vi "IP SETTING.vi"() -> ()   [LabVIEW 2017]
uses:
  <vilib>/addons/database/Connection.llb/DB Tools Open Connec (String).vi
  Global/Global 1.vi
  <vilib>/addons/database/NI_Database_API.lvlib
panel:
  in  "SAVE":bool
  in  "Cluster":T1
  out "error out":errorcluster
  in  "error in (no error)":errorcluster
  in  "EXIT":bool
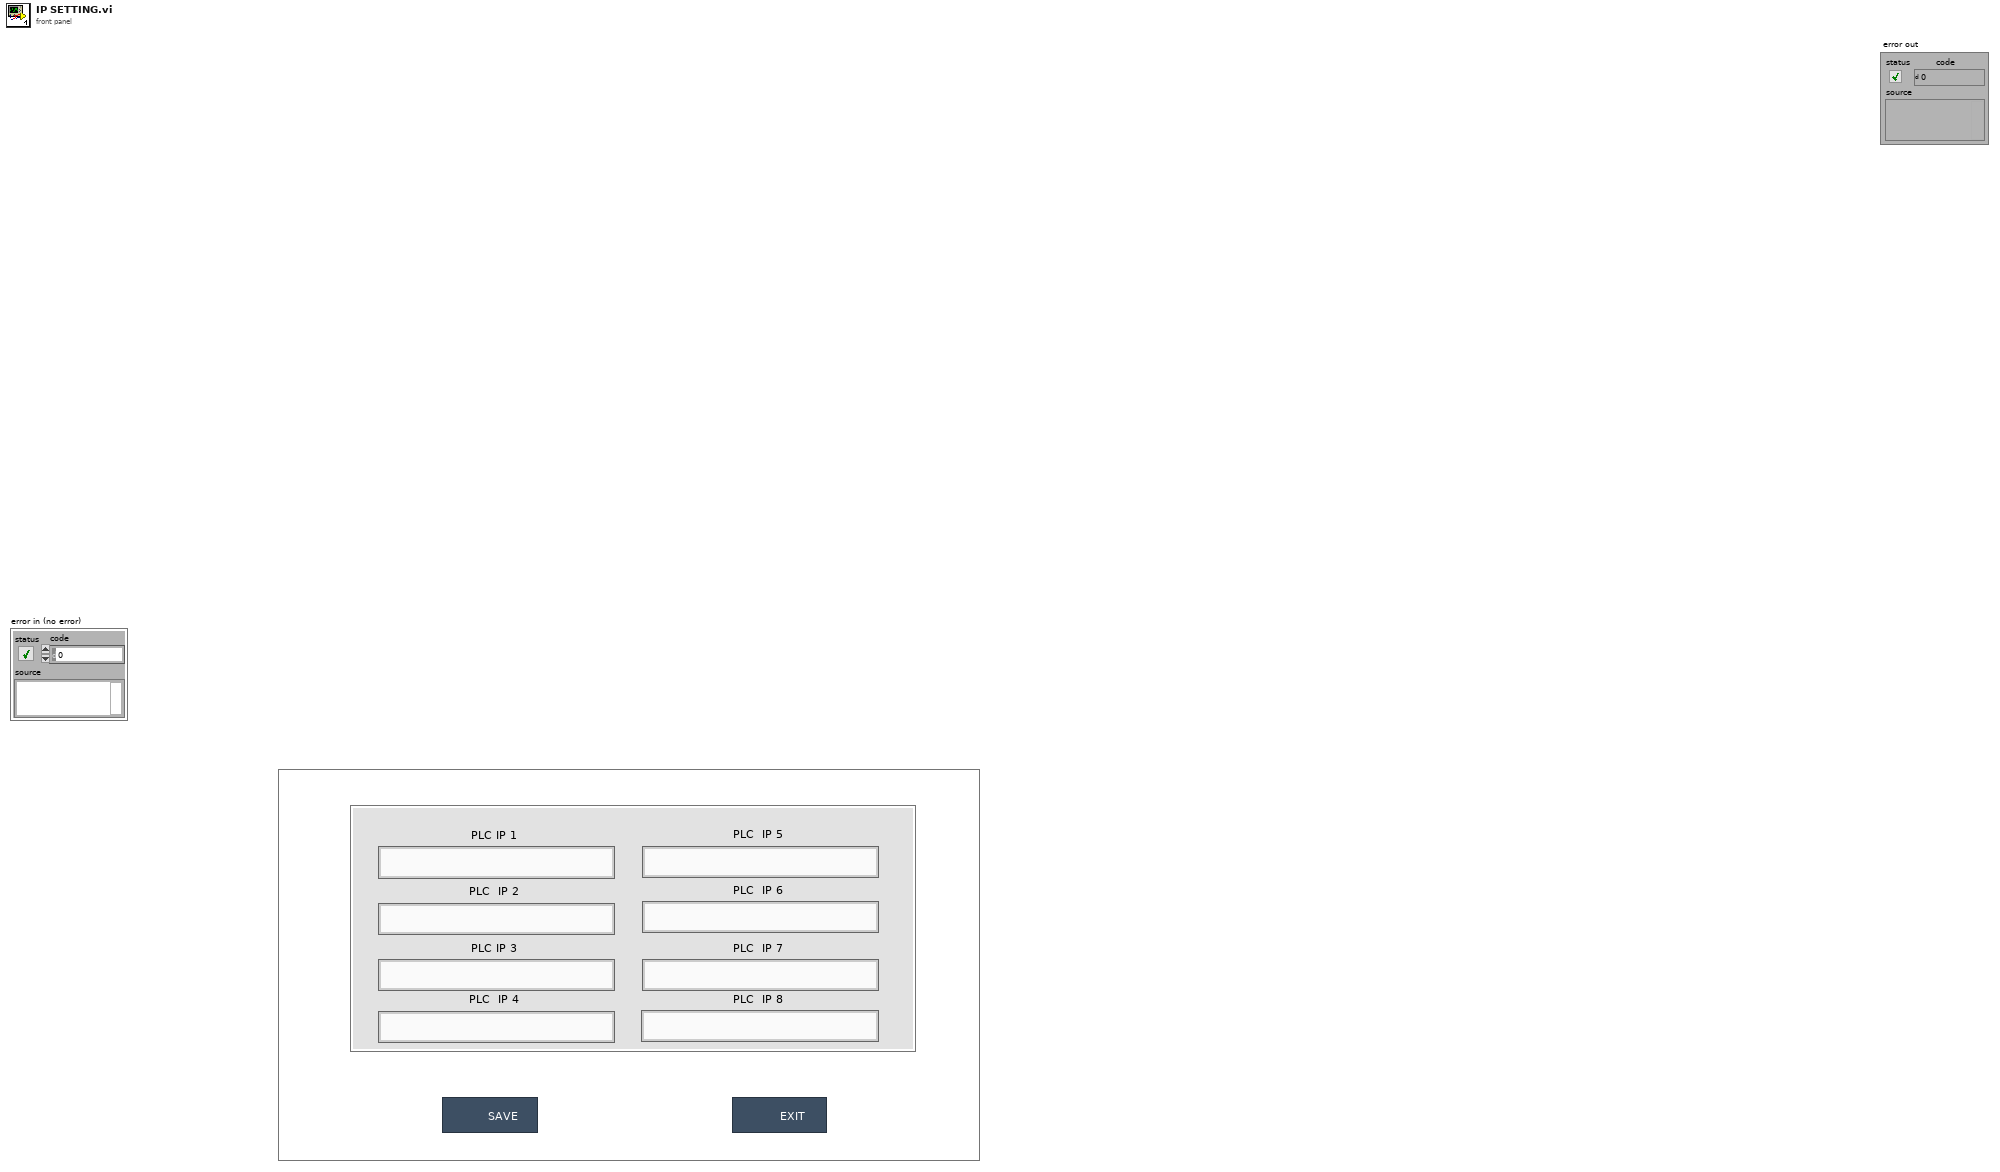
[diagram p1: front panel]
types:
  T1 = cluster{"PLC IP 1":string, "PLC  IP 2":string, "PLC IP 3":string, "PLC  IP 4":string, "PLC  IP 5":string, "PLC  IP 6":string, "PLC  IP 7":string, "PLC  IP 8":string}
  T2 = typedef "NI_Database_API.lvlib/Conn ObjectReference.ctl" = refnum<k1>
  T3 = enum32{"invalid app kind", "Development System", "Run Time System", "Student Edition", "Embedded LabVIEW", "Evaluation", "Custom"}
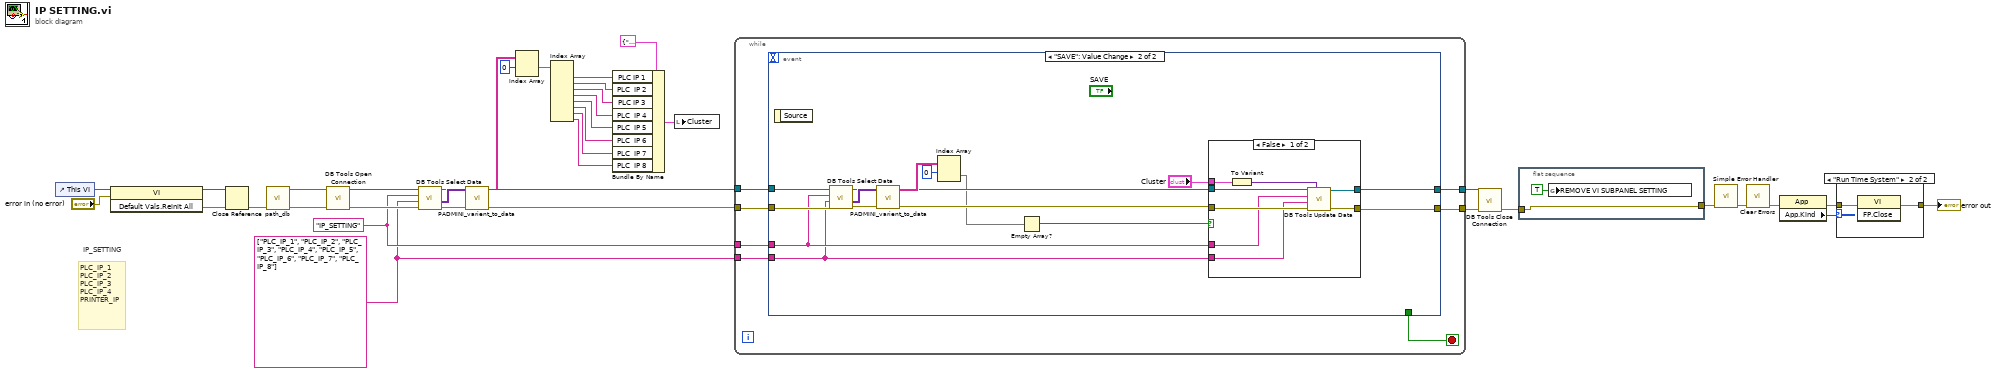
[diagram p0: block diagram]
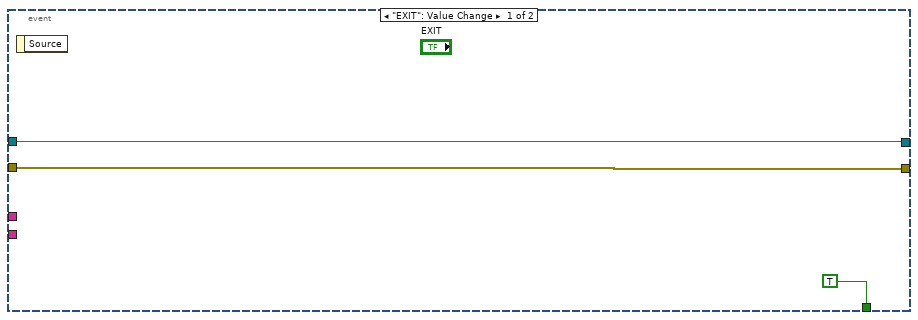
[diagram p2: hidden frame]
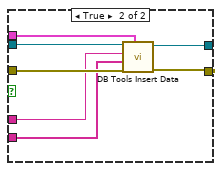
[diagram p3: hidden frame]
diagram:
  w8 = string[] ["PLC_IP_1", "PLC_IP_2", "PLC_IP_3", "PLC_IP_4", "PLC_IP_5", "PLC_IP_6", "PLC_IP_7", "PLC_IP_8"] ("columns")
  w13 = "IP_SETTING" ("table")
  # "PLC_IP_1\nPLC_IP_2\nPLC_IP_3\nPLC_IP_4\nPRINTER_IP"
  # "IP_SETTING"
  n1 = control-ref of="This VI"() -> (w37:refnum<vi>)
  n2 = invoke class="VI" method="Default Vals.Reinit All"(reference=w37, error in="error in (no error)") -> (reference out=w35:refnum<vi>, error out=w36:errorcluster)  [unwired: 1 in, 1 out]
  n3 = Close Reference(reference=w35, error in (no error)=w36) -> (error out=w27:errorcluster)
  n4 = call "path_db.vi"("error in"=w27) -> ("error out"=w21:errorcluster, "resulting string"=w26:string)  [unwired: 9 in]
  n5 = call-poly <vilib>:"DB Tools Open Connection.vi"("error in (no error)"=w21, "connection information"=w26) -> ("error out"=w25:errorcluster, "connection reference"=w24:T2)  [unwired: 6 in]
  n6 = call <vilib>:"DB Tools Select Data.vi"("error in (no error)"=w25, "columns"=w8, "table"=w13, "connection reference"=w24) -> ("error out"=w23:errorcluster, "data"=w22:variant[][], "connection reference out"=w16:T2)  [unwired: 2 in]
  n7 = call "PADMINI_varient_to_data.vi"("error in (no error)"=w23, "data"=w22) -> ("error out"=w20:errorcluster, "Array"=w15:string[][])  [unwired: 8 in]
  n8 = Index Array(array=w15, index (row)=0 ("disabled index (col)")) -> (element=w14:string[])  [unwired: 1 in]
  n9 = Index Array(array=w14) -> (element #1=w19:string, element #2=w18:string, element #3=w17:string, element #4=w7:string, element #5=w5:string, element #6=w4:string, element #7=w2:string, element #8=w1:string)  [unwired: 8 in]
  n10 = Bundle By Name(cluster=T1 {"PLC IP 1"="", "PLC  IP 2"="", "PLC IP 3"="", "PLC  IP 4"="", "PLC  IP 5"="", "PLC  IP 6"="", "PLC  IP 7"="", "PLC  IP 8"=""} ("Cluster"), "PLC IP 1"=w19, "PLC  IP 2"=w18, "PLC IP 3"=w17, "PLC  IP 4"=w7, "PLC  IP 5"=w5, "PLC  IP 6"=w4, "PLC  IP 7"=w2, "PLC  IP 8"=w1) -> (w6:T1)
  n11 = local write "Cluster"(w6) -> ()
  n12 = while {
    tunnel: [w43] -> w11
    tunnel: w20 -> [w44]
    tunnel: w16 -> [w41]
    tunnel: [w40] -> w12
    tunnel: w13 -> [w39]
    tunnel: w8 -> [w38]
    stop <- w42 stop-if-true
    n13 = event shown="[1] \"SAVE\": Value Change" {
      selector: _ -> [_ _]
      dyn-events: _ -> [_ _]
      timeout: _ -> [_ _]
      tunnel: w44 -> [w47 w54]
      tunnel: [w47 w62] -> w43
      tunnel: [TRUE _] -> w42
      tunnel: w41 -> [w45 w55]
      tunnel: [w45 w61] -> w40
      tunnel: w39 -> [_ w53]
      tunnel: w38 -> [_ w52]
      event "EXIT": Value Change {
        n14 = event-data() -> ()  [unwired: 1 in, 1 out]
      }
      event "SAVE": Value Change {
        n15 = event-data() -> ()  [unwired: 1 in, 1 out]
        n16 = call <vilib>:"DB Tools Select Data.vi"("error in (no error)"=w54, "columns"=w52, "table"=w53, "connection reference"=w55) -> ("error out"=w56:errorcluster, "data"=w57:variant[][], "connection reference out"=w50:T2)  [unwired: 2 in]
        n17 = call "PADMINI_varient_to_data.vi"("error in (no error)"=w56, "data"=w57) -> ("error out"=w51:errorcluster, "Array"=w58:string[][])  [unwired: 8 in]
        n18 = Index Array(array=w58, index (row)=0 ("disabled index (col)")) -> (element=w49:string[])  [unwired: 1 in]
        n19 = Empty Array?(array=w49) -> (empty?=w48:bool)
        n20 = case shown="False" w48 {
          tunnel: w51 -> [w69 w77]
          tunnel: w50 -> [w70 w75]
          tunnel: [w67 w76] -> w62
          tunnel: [w68 w74] -> w61
          tunnel: w53 -> [w66 w73]
          tunnel: w52 -> [w65 w72]
          tunnel: "Cluster" -> [w64 w71]
          frame False {
            n21 = To Variant(anything=w64) -> (Variant=w63:variant)
            n22 = call <vilib>:"DB Tools Update Data.vi"("data"=w63, "error in (no error)"=w69, "columns"=w65, "table"=w66, "connection reference"=w70) -> ("error out"=w67:errorcluster, "connection reference out"=w68:T2)  [unwired: 5 in]
          }
          frame True {
            n23 = call <vilib>:"DB Tools Insert Data.vi"("data"=w71, "error in (no error)"=w77, "columns"=w72, "table"=w73, "connection reference"=w75) -> ("error out"=w76:errorcluster, "connection reference out"=w74:T2)  [unwired: 5 in]
          }
        }
      }
    }
  }
  n24 = call <vilib>:"DB Tools Close Connection.vi"("error in (no error)"=w11, "connection reference"=w12) -> ("error out"=w10:errorcluster)  [unwired: 5 in]
  n25 = flat-sequence {
    tunnel: w10 -> [w79]
    tunnel: [w79] -> w28
    frame #0 {
      n26 = global write "Global 1.vi" "REMOVE VI SUBPANEL SETTING"(TRUE ("REMOVE_VI _SUBPANEL_3")) -> ()
    }
  }
  n27 = call <vilib>:"Simple Error Handler.vi"("error in (no error)"=w28) -> ("error out"=w33:errorcluster)  [unwired: 4 in, 4 out]
  n28 = call <vilib>:"Clear Errors.vi"("error in (no error)"=w33) -> ("error out"=w30:errorcluster)  [unwired: 5 in, 1 out]
  n29 = property class="App"(error in=w30) -> (error out=w31:errorcluster, "App.Kind"=w32:T3)  [unwired: 1 in, 1 out]
  n30 = case shown="\"Run Time System\"" w32 {
    tunnel: w31 -> [w80 w82]
    tunnel: [w80 w81] -> w29
    frame Default {
    }
    frame "Run Time System" {
      n31 = invoke class="VI" method="FP.Close"(error in=w82) -> (error out=w81:errorcluster)  [unwired: 2 in, 2 out]
    }
  }
  "error out" <- w29
